vi "Time_to_word.vi"(4 "Tempo (sec)":u16) -> (1 "word":u16)   [LabVIEW 2022 SP3]
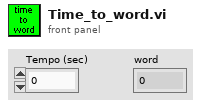
[diagram p1: front panel]
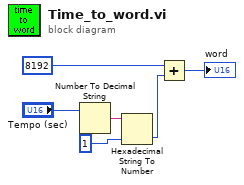
[diagram p0: block diagram]
diagram:
  n1 = Number To Decimal String(number="Tempo (sec)") -> (decimal integer string=w6:string)  [unwired: 1 in]
  n2 = Hexadecimal String To Number(string=w6, default (0uL)=u16 1 ("default (0 U32)")) -> (number=w4:u16)  [unwired: 1 in, 1 out]
  n3 = Add(x=u16 8192 ("number 2"), y=w4) -> (x+y=→"word":u16)
